vi "Double to Exact String.vi"(8 "Error In":errorcluster, 10 "Numeric Control":dbl format="%#.10g") -> (0 "Error Out":errorcluster, 2 "F-format string":string)   [LabVIEW 2016]
doc: "This VI takes a double and convert it to a string. Also output the correct number of digits after the decimal point based on the string precision."
uses:
  <vilib>/regexp/Match Regular Expression.xnode
panel:
  out "after match":string
  out "Display Format:Precision":u8
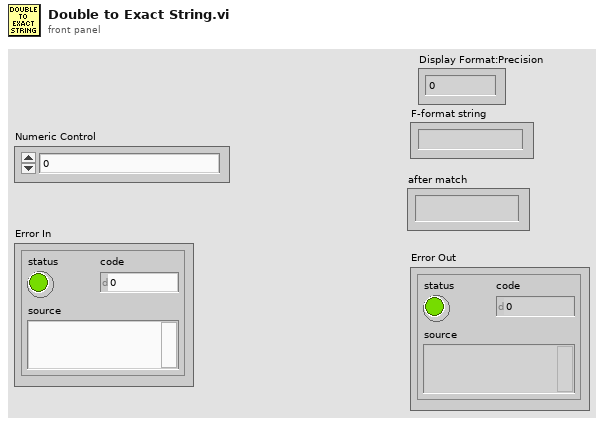
[diagram p1: front panel]
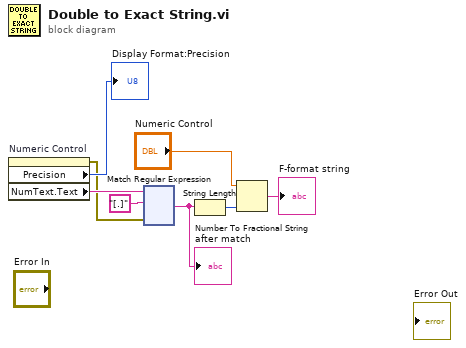
[diagram p0: block diagram]
diagram:
  n1 = property on="Numeric Control" class="DigNum (strict)"() -> (error out=w1:errorcluster, "Precision"=→"Display Format:Precision":u8, "NumText.Text"=w4:string)  [unwired: 2 in, 1 out]
  n2 = xnode "Match Regular Expression"("input string"=w4, "regular expression"="[.]", "error in"=w1) -> ("after match"=w3:string)  [unwired: 3 in, 4 out]
  "after match" <- w3
  n3 = String Length(string=w3) -> (length=w2:i32)
  n4 = Number To Fractional String(number="Numeric Control", precision (6)=w2) -> (F-format string=→"F-format string":string)  [unwired: 2 in]
